vi "TH2829_Analysis_Data.vi"(0 "字符串":string) -> (14 "Turns Result":sgl[][](array[numeric]) format="%#_6f", 15 "Lx Result":sgl[][](array[numeric]) format="%#_6f", 16 "Lk Result":sgl[][](array[numeric]) format="%#_6f", 17 "DCR Result":sgl[][](array[numeric]) format="%#_6f")   [LabVIEW 2018]
panel:
  out "LED IrCompare Result":u8[][](array[numeric])
  out "LED VfCompare Result":u8[][](array[numeric])
  out "LED IrResult":sgl[][](array[numeric]) format="%#_6f"
  out "LED VfResult":sgl[][](array[numeric]) format="%#_6f"
  out "Bls Result":sgl[][](array[numeric]) format="%#_6f"
  out "总判断":u8
  out "PS Compare Result":u8[][](array[numeric])
  out "Balance Compare Result":u8[][](array[numeric])
  out "Z Compare Result":u8[][](array[numeric])
  out "Rs Compare Result":u8[][](array[numeric])
  out "LxQ Compare Result":u8[][](array[numeric])
  out "DCR Compare Result":u8[][](array[numeric])
  out "C Compare Result":u8[][](array[numeric])
  out "Lk Compare Result":u8[][](array[numeric])
  out "Lx Compare Result":u8[][](array[numeric])
  out "Turns Compare Result":u8[][](array[numeric])
  out "Polarity Result1":string[][](array[string])
  out "Polarity Result":u8[][](array[numeric])
  out "Zx Result":sgl[][](array[numeric]) format="%#_6f"
  out "ACR Result":sgl[][](array[numeric]) format="%#_6f"
  out "LxQ Result":sgl[][](array[numeric]) format="%#_6f"
  out "Cx Result":sgl[][](array[numeric]) format="%#_6f"
  out "Primary Sets":string
  out "head":string
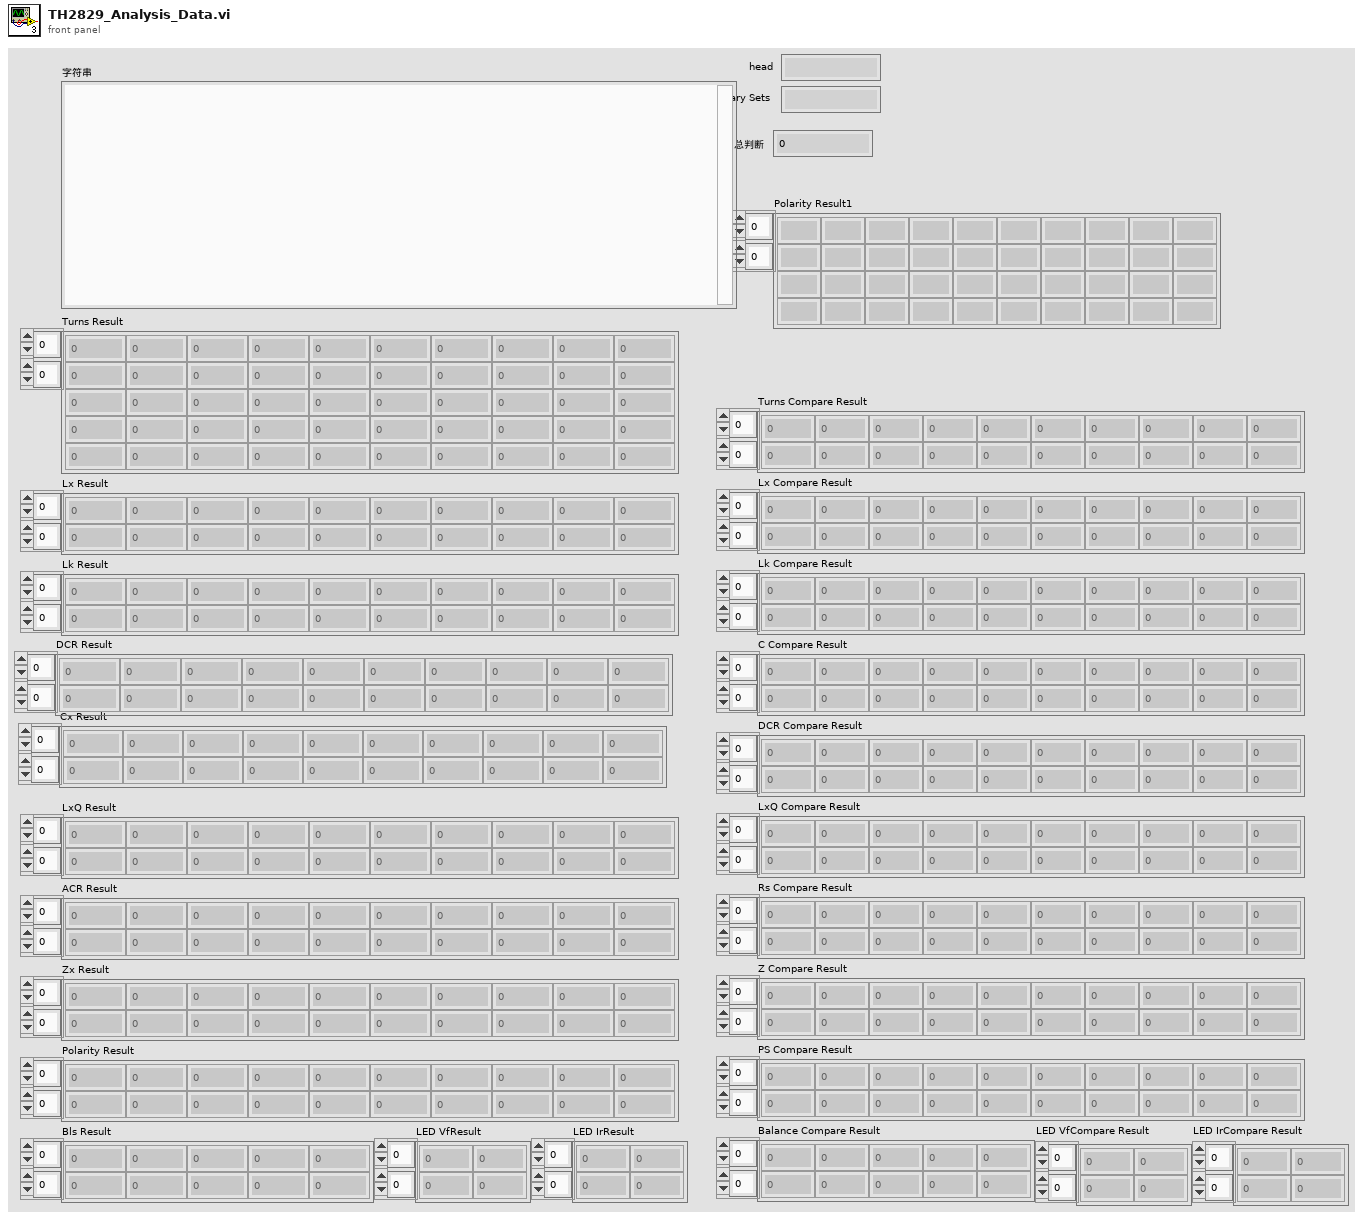
[diagram p1: front panel]
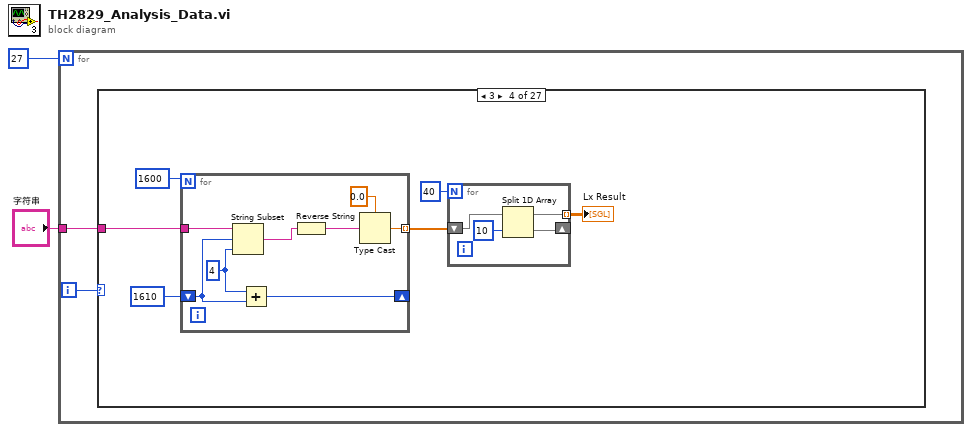
[diagram p0: block diagram]
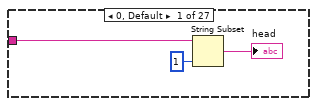
[diagram p2: hidden frame]
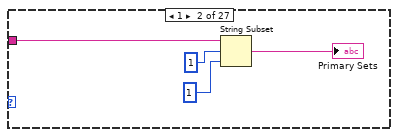
[diagram p3: hidden frame]
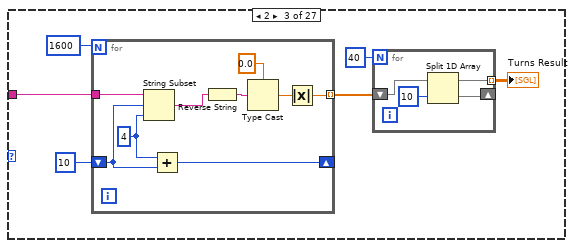
[diagram p4: hidden frame]
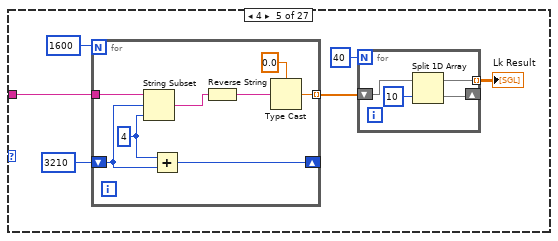
[diagram p5: hidden frame]
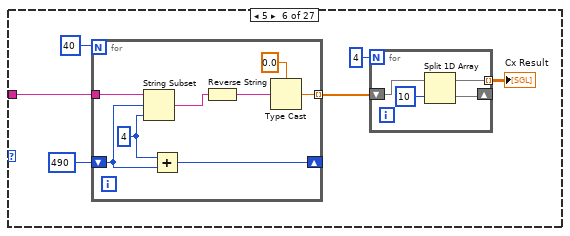
[diagram p6: hidden frame]
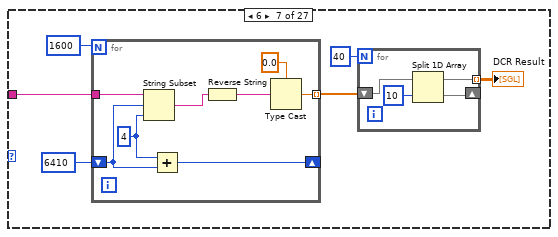
[diagram p7: hidden frame]
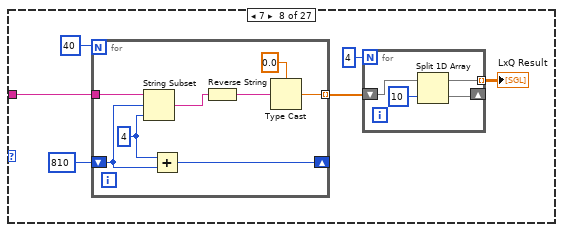
[diagram p8: hidden frame]
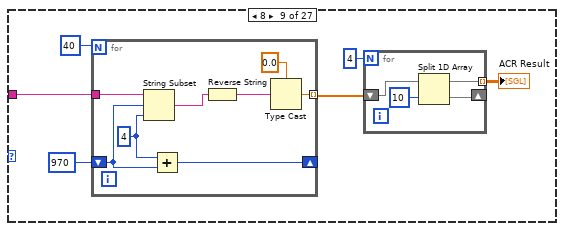
[diagram p9: hidden frame]
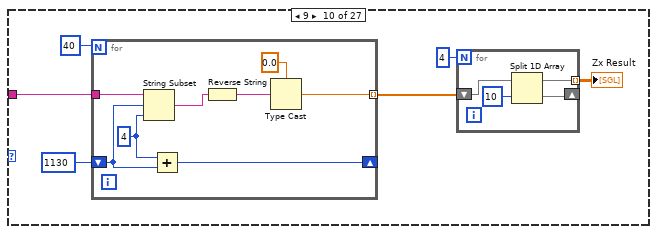
[diagram p10: hidden frame]
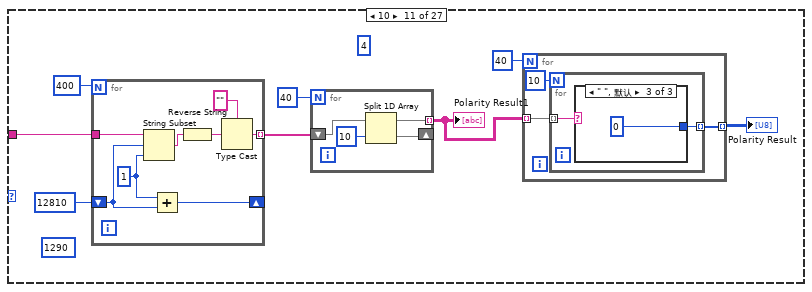
[diagram p11: hidden frame]
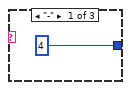
[diagram p12: hidden frame]
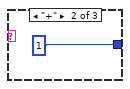
[diagram p13: hidden frame]
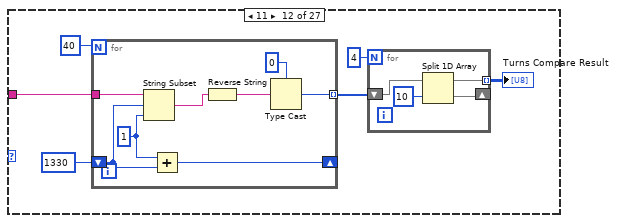
[diagram p14: hidden frame]
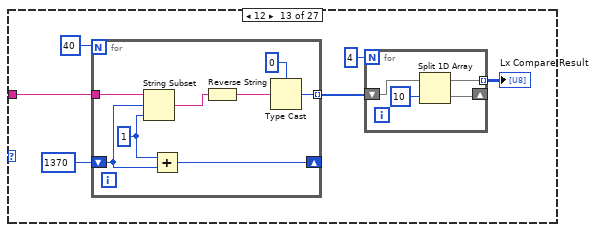
[diagram p15: hidden frame]
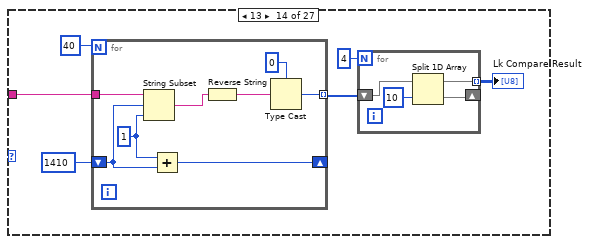
[diagram p16: hidden frame]
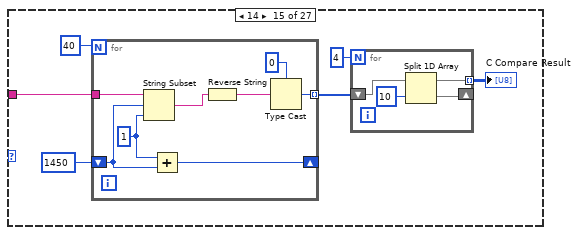
[diagram p17: hidden frame]
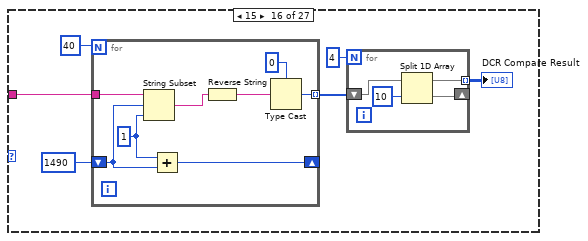
[diagram p18: hidden frame]
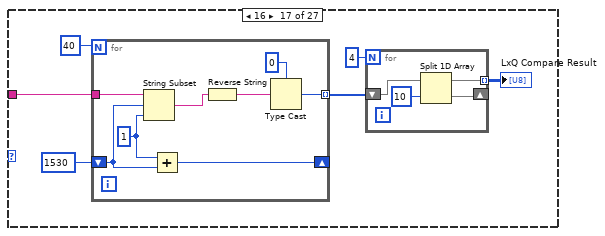
[diagram p19: hidden frame]
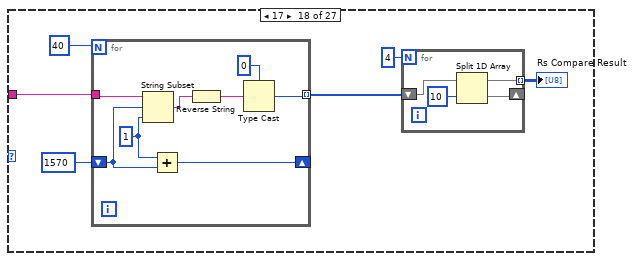
[diagram p20: hidden frame]
diagram:
  n1 = for {
    N: 27 -> [_]
    tunnel: "字符串" -> [w3]
    i -> [w4]
    n2 = case shown="3" w4 {
      tunnel: w3 -> [w7 w11 w16 w35 w53 w71 w89 w107 w125 w143 w163 w189 w207 w225 w243 w261 w279 w297 w315 w333 w351 w368 w372 w390 w408 w426 w444]
      frame 0, Default {
        n3 = String Subset(string=w7, length (rest)=1 ("长度（剩余）")) -> (substring=→"head":string)  [unwired: 1 in]
      }
      frame 1 {
        n4 = String Subset ("截取字符串")(string=w11, offset (0)=1 ("长度（剩余）"), length (rest)=1 ("长度（剩余）")) -> (substring=→"Primary Sets":string)
      }
      frame 2 {
        n5 = for {
          N: 1600 -> [_]
          shift-right: [w26] -> _
          shift-left: 10 ("长度（剩余）") -> [w22]
          tunnel: w16 -> [w21]
          tunnel: [w18] -> w14 mode=indexing
          w23 = 4 ("长度（剩余）")
          n6 = String Subset(string=w21, offset (0)=w22, length (rest)=w23) -> (substring=w20:string)
          n7 = Add(x=w23, y=w22) -> (x+y=w26:i32)
          n8 = Reverse String(1:w20) -> (0:w25:string)
          n9 = Type Cast(type=sgl 0.0 ("长度（剩余）"), x=w25) -> (*(type *) &x=w19:sgl)
          n10 = Absolute Value(x=w19) -> (abs(x)=w18:sgl)
        }
        n11 = for {
          N: 40 -> [_]
          shift-right: [w29] -> _
          shift-left: w14 -> [w27]
          tunnel: [w28] -> w12 mode=indexing
          n12 = Split 1D Array(array=w27, index=10 ("索引")) -> (first subarray=w28:sgl[], second subarray=w29:sgl[])
        }
        "Turns Result" <- w12
      }
      frame 3 {
        n13 = for {
          N: 1600 -> [_]
          shift-right: [w44] -> _
          shift-left: 1610 ("长度（剩余）") -> [w40]
          tunnel: w35 -> [w39]
          tunnel: [w37] -> w33 mode=indexing
          w41 = 4 ("长度（剩余）")
          n14 = String Subset(string=w39, offset (0)=w40, length (rest)=w41) -> (substring=w38:string)
          n15 = Add(x=w41, y=w40) -> (x+y=w44:i32)
          n16 = Reverse String(1:w38) -> (0:w43:string)
          n17 = Type Cast(type=sgl 0.0 ("长度（剩余）"), x=w43) -> (*(type *) &x=w37:sgl)
        }
        n18 = for {
          N: 40 -> [_]
          shift-right: [w47] -> _
          shift-left: w33 -> [w45]
          tunnel: [w46] -> w31 mode=indexing
          n19 = Split 1D Array(array=w45, index=10 ("索引")) -> (first subarray=w46:sgl[], second subarray=w47:sgl[])
        }
        "Lx Result" <- w31
      }
      frame 4 {
        n20 = for {
          N: 1600 -> [_]
          shift-right: [w62] -> _
          shift-left: 3210 ("长度（剩余）") -> [w58]
          tunnel: w53 -> [w57]
          tunnel: [w55] -> w51 mode=indexing
          w59 = 4 ("长度（剩余）")
          n21 = String Subset(string=w57, offset (0)=w58, length (rest)=w59) -> (substring=w56:string)
          n22 = Add(x=w59, y=w58) -> (x+y=w62:i32)
          n23 = Reverse String(1:w56) -> (0:w61:string)
          n24 = Type Cast(type=sgl 0.0 ("长度（剩余）"), x=w61) -> (*(type *) &x=w55:sgl)
        }
        n25 = for {
          N: 40 -> [_]
          shift-right: [w65] -> _
          shift-left: w51 -> [w63]
          tunnel: [w64] -> w49 mode=indexing
          n26 = Split 1D Array(array=w63, index=10 ("索引")) -> (first subarray=w64:sgl[], second subarray=w65:sgl[])
        }
        "Lk Result" <- w49
      }
      frame 5 {
        n27 = for {
          N: 40 -> [_]
          shift-right: [w80] -> _
          shift-left: 490 ("长度（剩余）") -> [w76]
          tunnel: w71 -> [w75]
          tunnel: [w73] -> w69 mode=indexing
          w77 = 4 ("长度（剩余）")
          n28 = String Subset(string=w75, offset (0)=w76, length (rest)=w77) -> (substring=w74:string)
          n29 = Add(x=w77, y=w76) -> (x+y=w80:i32)
          n30 = Reverse String(1:w74) -> (0:w79:string)
          n31 = Type Cast(type=sgl 0.0 ("长度（剩余）"), x=w79) -> (*(type *) &x=w73:sgl)
        }
        n32 = for {
          N: 4 -> [_]
          shift-right: [w83] -> _
          shift-left: w69 -> [w81]
          tunnel: [w82] -> w67 mode=indexing
          n33 = Split 1D Array(array=w81, index=10 ("索引")) -> (first subarray=w82:sgl[], second subarray=w83:sgl[])
        }
        "Cx Result" <- w67
      }
      frame 6 {
        n34 = for {
          N: 1600 -> [_]
          shift-right: [w98] -> _
          shift-left: 6410 ("长度（剩余）") -> [w94]
          tunnel: w89 -> [w93]
          tunnel: [w91] -> w87 mode=indexing
          w95 = 4 ("长度（剩余）")
          n35 = String Subset(string=w93, offset (0)=w94, length (rest)=w95) -> (substring=w92:string)
          n36 = Add(x=w95, y=w94) -> (x+y=w98:i32)
          n37 = Reverse String(1:w92) -> (0:w97:string)
          n38 = Type Cast(type=sgl 0.0 ("长度（剩余）"), x=w97) -> (*(type *) &x=w91:sgl)
        }
        n39 = for {
          N: 40 -> [_]
          shift-right: [w101] -> _
          shift-left: w87 -> [w99]
          tunnel: [w100] -> w85 mode=indexing
          n40 = Split 1D Array(array=w99, index=10 ("索引")) -> (first subarray=w100:sgl[], second subarray=w101:sgl[])
        }
        "DCR Result" <- w85
      }
      frame 7 {
        n41 = for {
          N: 40 -> [_]
          shift-right: [w116] -> _
          shift-left: 810 ("长度（剩余）") -> [w112]
          tunnel: w107 -> [w111]
          tunnel: [w109] -> w105 mode=indexing
          w113 = 4 ("长度（剩余）")
          n42 = String Subset(string=w111, offset (0)=w112, length (rest)=w113) -> (substring=w110:string)
          n43 = Add(x=w113, y=w112) -> (x+y=w116:i32)
          n44 = Reverse String(1:w110) -> (0:w115:string)
          n45 = Type Cast(type=sgl 0.0 ("长度（剩余）"), x=w115) -> (*(type *) &x=w109:sgl)
        }
        n46 = for {
          N: 4 -> [_]
          shift-right: [w119] -> _
          shift-left: w105 -> [w117]
          tunnel: [w118] -> w103 mode=indexing
          n47 = Split 1D Array(array=w117, index=10 ("索引")) -> (first subarray=w118:sgl[], second subarray=w119:sgl[])
        }
        "LxQ Result" <- w103
      }
      frame 8 {
        n48 = for {
          N: 40 -> [_]
          shift-right: [w134] -> _
          shift-left: 970 ("长度（剩余）") -> [w130]
          tunnel: w125 -> [w129]
          tunnel: [w127] -> w123 mode=indexing
          w131 = 4 ("长度（剩余）")
          n49 = String Subset(string=w129, offset (0)=w130, length (rest)=w131) -> (substring=w128:string)
          n50 = Add(x=w131, y=w130) -> (x+y=w134:i32)
          n51 = Reverse String(1:w128) -> (0:w133:string)
          n52 = Type Cast(type=sgl 0.0 ("长度（剩余）"), x=w133) -> (*(type *) &x=w127:sgl)
        }
        n53 = for {
          N: 4 -> [_]
          shift-right: [w137] -> _
          shift-left: w123 -> [w135]
          tunnel: [w136] -> w121 mode=indexing
          n54 = Split 1D Array(array=w135, index=10 ("索引")) -> (first subarray=w136:sgl[], second subarray=w137:sgl[])
        }
        "ACR Result" <- w121
      }
      frame 9 {
        n55 = for {
          N: 40 -> [_]
          shift-right: [w152] -> _
          shift-left: 1130 ("长度（剩余）") -> [w148]
          tunnel: w143 -> [w147]
          tunnel: [w145] -> w141 mode=indexing
          w149 = 4 ("长度（剩余）")
          n56 = String Subset(string=w147, offset (0)=w148, length (rest)=w149) -> (substring=w146:string)
          n57 = Add(x=w149, y=w148) -> (x+y=w152:i32)
          n58 = Reverse String(1:w146) -> (0:w151:string)
          n59 = Type Cast(type=sgl 0.0 ("长度（剩余）"), x=w151) -> (*(type *) &x=w145:sgl)
        }
        n60 = for {
          N: 4 -> [_]
          shift-right: [w155] -> _
          shift-left: w141 -> [w153]
          tunnel: [w154] -> w139 mode=indexing
          n61 = Split 1D Array(array=w153, index=10 ("索引")) -> (first subarray=w154:sgl[], second subarray=w155:sgl[])
        }
        "Zx Result" <- w139
      }
      frame 10 {
        (unwired) 1290 ("长度（剩余）")
        (unwired) 4
        n62 = for {
          N: 400 -> [_]
          shift-right: [w180] -> _
          shift-left: 12810 ("长度（剩余）") -> [w177]
          tunnel: w163 -> [w176]
          tunnel: [w174] -> w158 mode=indexing
          w178 = 1 ("长度（剩余）")
          n63 = String Subset(string=w176, offset (0)=w177, length (rest)=w178) -> (substring=w175:string)
          n64 = Add(x=w178, y=w177) -> (x+y=w180:i32)
          n65 = Reverse String(1:w175) -> (0:w179:string)
          n66 = Type Cast(type="", x=w179) -> (*(type *) &x=w174:string)
        }
        n67 = for {
          N: 40 -> [_]
          shift-right: [w183] -> _
          shift-left: w158 -> [w181]
          tunnel: [w182] -> w157 mode=indexing
          n68 = Split 1D Array(array=w181, index=10 ("索引")) -> (first subarray=w182:string[], second subarray=w183:string[])
        }
        "Polarity Result1" <- w157
        n69 = for {
          N: 40 -> [_]
          tunnel: w157 -> [w166] mode=indexing
          tunnel: [w165] -> w159 mode=indexing
          n70 = for {
            N: 10 -> [_]
            tunnel: w166 -> [w169] mode=indexing
            tunnel: [w168] -> w165 mode=indexing
            n71 = case shown="\" \", 默认" w169 {
              tunnel: [u8 4 u8 1 u8 0] -> w168
              frame "-" {
              }
              frame "+" {
              }
              frame " ", Default {
              }
            }
          }
        }
        "Polarity Result" <- w159
      }
      frame 11 {
        n72 = for {
          N: 40 -> [_]
          shift-right: [w198] -> _
          shift-left: 1330 ("长度（剩余）") -> [w194]
          tunnel: w189 -> [w193]
          tunnel: [w191] -> w187 mode=indexing
          w195 = 1 ("长度（剩余）")
          n73 = String Subset ("截取字符串")(string=w193, offset (0)=w194, length (rest)=w195) -> (substring=w192:string)
          n74 = Add(x=w195, y=w194) -> (x+y=w198:i32)
          n75 = Reverse String(1:w192) -> (0:w197:string)
          n76 = Type Cast(type=u8 0 ("长度（剩余）"), x=w197) -> (*(type *) &x=w191:u8)
        }
        n77 = for {
          N: 4 -> [_]
          shift-right: [w201] -> _
          shift-left: w187 -> [w199]
          tunnel: [w200] -> w185 mode=indexing
          n78 = Split 1D Array(array=w199, index=10 ("索引")) -> (first subarray=w200:u8[], second subarray=w201:u8[])
        }
        "Turns Compare Result" <- w185
      }
      frame 12 {
        n79 = for {
          N: 40 -> [_]
          shift-right: [w216] -> _
          shift-left: 1370 ("长度（剩余）") -> [w212]
          tunnel: w207 -> [w211]
          tunnel: [w209] -> w205 mode=indexing
          w213 = 1 ("长度（剩余）")
          n80 = String Subset(string=w211, offset (0)=w212, length (rest)=w213) -> (substring=w210:string)
          n81 = Add(x=w213, y=w212) -> (x+y=w216:i32)
          n82 = Reverse String(1:w210) -> (0:w215:string)
          n83 = Type Cast(type=u8 0 ("长度（剩余）"), x=w215) -> (*(type *) &x=w209:u8)
        }
        n84 = for {
          N: 4 -> [_]
          shift-right: [w219] -> _
          shift-left: w205 -> [w217]
          tunnel: [w218] -> w203 mode=indexing
          n85 = Split 1D Array(array=w217, index=10 ("索引")) -> (first subarray=w218:u8[], second subarray=w219:u8[])
        }
        "Lx Compare Result" <- w203
      }
      frame 13 {
        n86 = for {
          N: 40 -> [_]
          shift-right: [w234] -> _
          shift-left: 1410 ("长度（剩余）") -> [w230]
          tunnel: w225 -> [w229]
          tunnel: [w227] -> w223 mode=indexing
          w231 = 1 ("长度（剩余）")
          n87 = String Subset(string=w229, offset (0)=w230, length (rest)=w231) -> (substring=w228:string)
          n88 = Add(x=w231, y=w230) -> (x+y=w234:i32)
          n89 = Reverse String(1:w228) -> (0:w233:string)
          n90 = Type Cast(type=u8 0 ("长度（剩余）"), x=w233) -> (*(type *) &x=w227:u8)
        }
        n91 = for {
          N: 4 -> [_]
          shift-right: [w237] -> _
          shift-left: w223 -> [w235]
          tunnel: [w236] -> w221 mode=indexing
          n92 = Split 1D Array(array=w235, index=10 ("索引")) -> (first subarray=w236:u8[], second subarray=w237:u8[])
        }
        "Lk Compare Result" <- w221
      }
      frame 14 {
        n93 = for {
          N: 40 -> [_]
          shift-right: [w252] -> _
          shift-left: 1450 ("长度（剩余）") -> [w248]
          tunnel: w243 -> [w247]
          tunnel: [w245] -> w241 mode=indexing
          w249 = 1 ("长度（剩余）")
          n94 = String Subset(string=w247, offset (0)=w248, length (rest)=w249) -> (substring=w246:string)
          n95 = Add(x=w249, y=w248) -> (x+y=w252:i32)
          n96 = Reverse String(1:w246) -> (0:w251:string)
          n97 = Type Cast(type=u8 0 ("长度（剩余）"), x=w251) -> (*(type *) &x=w245:u8)
        }
        n98 = for {
          N: 4 -> [_]
          shift-right: [w255] -> _
          shift-left: w241 -> [w253]
          tunnel: [w254] -> w239 mode=indexing
          n99 = Split 1D Array(array=w253, index=10 ("索引")) -> (first subarray=w254:u8[], second subarray=w255:u8[])
        }
        "C Compare Result" <- w239
      }
      frame 15 {
        n100 = for {
          N: 40 -> [_]
          shift-right: [w270] -> _
          shift-left: 1490 ("长度（剩余）") -> [w266]
          tunnel: w261 -> [w265]
          tunnel: [w263] -> w259 mode=indexing
          w267 = 1 ("长度（剩余）")
          n101 = String Subset(string=w265, offset (0)=w266, length (rest)=w267) -> (substring=w264:string)
          n102 = Add(x=w267, y=w266) -> (x+y=w270:i32)
          n103 = Reverse String(1:w264) -> (0:w269:string)
          n104 = Type Cast(type=u8 0 ("长度（剩余）"), x=w269) -> (*(type *) &x=w263:u8)
        }
        n105 = for {
          N: 4 -> [_]
          shift-right: [w273] -> _
          shift-left: w259 -> [w271]
          tunnel: [w272] -> w257 mode=indexing
          n106 = Split 1D Array(array=w271, index=10 ("索引")) -> (first subarray=w272:u8[], second subarray=w273:u8[])
        }
        "DCR Compare Result" <- w257
      }
      frame 16 {
        n107 = for {
          N: 40 -> [_]
          shift-right: [w288] -> _
          shift-left: 1530 ("长度（剩余）") -> [w284]
          tunnel: w279 -> [w283]
          tunnel: [w281] -> w277 mode=indexing
          w285 = 1 ("长度（剩余）")
          n108 = String Subset(string=w283, offset (0)=w284, length (rest)=w285) -> (substring=w282:string)
          n109 = Add(x=w285, y=w284) -> (x+y=w288:i32)
          n110 = Reverse String(1:w282) -> (0:w287:string)
          n111 = Type Cast(type=u8 0 ("长度（剩余）"), x=w287) -> (*(type *) &x=w281:u8)
        }
        n112 = for {
          N: 4 -> [_]
          shift-right: [w291] -> _
          shift-left: w277 -> [w289]
          tunnel: [w290] -> w275 mode=indexing
          n113 = Split 1D Array(array=w289, index=10 ("索引")) -> (first subarray=w290:u8[], second subarray=w291:u8[])
        }
        "LxQ Compare Result" <- w275
      }
      frame 17 {
        n114 = for {
          N: 40 -> [_]
          shift-right: [w306] -> _
          shift-left: 1570 ("长度（剩余）") -> [w300]
          tunnel: w297 -> [w301]
          tunnel: [w302] -> w295 mode=indexing
          w299 = 1 ("长度（剩余）")
          n115 = String Subset(string=w301, offset (0)=w300, length (rest)=w299) -> (substring=w303:string)
          n116 = Add(x=w299, y=w300) -> (x+y=w306:i32)
          n117 = Reverse String(1:w303) -> (0:w305:string)
          n118 = Type Cast(type=u8 0 ("长度（剩余）"), x=w305) -> (*(type *) &x=w302:u8)
        }
        n119 = for {
          N: 4 -> [_]
          shift-right: [w309] -> _
          shift-left: w295 -> [w307]
          tunnel: [w308] -> w293 mode=indexing
          n120 = Split 1D Array(array=w307, index=10 ("索引")) -> (first subarray=w308:u8[], second subarray=w309:u8[])
        }
        "Rs Compare Result" <- w293
      }
      frame 18 {
        n121 = for {
          N: 40 -> [_]
          shift-right: [w324] -> _
          shift-left: 1610 ("长度（剩余）") -> [w318]
          tunnel: w315 -> [w319]
          tunnel: [w320] -> w313 mode=indexing
          w317 = 1 ("长度（剩余）")
          n122 = Add(x=w317, y=w318) -> (x+y=w324:i32)
          n123 = String Subset(string=w319, offset (0)=w318, length (rest)=w317) -> (substring=w321:string)
          n124 = Reverse String(1:w321) -> (0:w323:string)
          n125 = Type Cast(type=u8 0 ("长度（剩余）"), x=w323) -> (*(type *) &x=w320:u8)
        }
        n126 = for {
          N: 4 -> [_]
          shift-right: [w327] -> _
          shift-left: w313 -> [w325]
          tunnel: [w326] -> w311 mode=indexing
          n127 = Split 1D Array(array=w325, index=10 ("索引")) -> (first subarray=w326:u8[], second subarray=w327:u8[])
        }
        "Z Compare Result" <- w311
      }
      frame 19 {
        n128 = for {
          N: 40 -> [_]
          shift-right: [w342] -> _
          shift-left: 1650 ("长度（剩余）") -> [w337]
          tunnel: w333 -> [w338]
          tunnel: [w339] -> w331 mode=indexing
          w336 = 1 ("长度（剩余）")
          n129 = String Subset(string=w338, offset (0)=w337, length (rest)=w336) -> (substring=w340:string)
          n130 = Add(x=w336, y=w337) -> (x+y=w342:i32)
          n131 = Reverse String(1:w340) -> (0:w341:string)
          n132 = Type Cast(type=u8 0 ("长度（剩余）"), x=w341) -> (*(type *) &x=w339:u8)
        }
        n133 = for {
          N: 4 -> [_]
          shift-right: [w345] -> _
          shift-left: w331 -> [w343]
          tunnel: [w344] -> w329 mode=indexing
          n134 = Split 1D Array(array=w343, index=10 ("索引")) -> (first subarray=w344:u8[], second subarray=w345:u8[])
        }
        "Balance Compare Result" <- w329
      }
      frame 20 {
        n135 = for {
          N: 40 -> [_]
          shift-right: [w360] -> _
          shift-left: 1690 ("长度（剩余）") -> [w355]
          tunnel: w351 -> [w356]
          tunnel: [w357] -> w349 mode=indexing
          w354 = 1 ("长度（剩余）")
          n136 = String Subset(string=w356, offset (0)=w355, length (rest)=w354) -> (substring=w358:string)
          n137 = Add(x=w354, y=w355) -> (x+y=w360:i32)
          n138 = Reverse String(1:w358) -> (0:w359:string)
          n139 = Type Cast(type=u8 0 ("长度（剩余）"), x=w359) -> (*(type *) &x=w357:u8)
        }
        n140 = for {
          N: 4 -> [_]
          shift-right: [w363] -> _
          shift-left: w349 -> [w361]
          tunnel: [w362] -> w347 mode=indexing
          n141 = Split 1D Array(array=w361, index=10 ("索引")) -> (first subarray=w362:u8[], second subarray=w363:u8[])
        }
        "PS Compare Result" <- w347
      }
      frame 21 {
        n142 = String Subset(string=w368, offset (0)=1730 ("长度（剩余）"), length (rest)=1 ("长度（剩余）")) -> (substring=w371:string)
        n143 = Reverse String(1:w371) -> (0:w369:string)
        n144 = Type Cast(type=u8 0 ("长度（剩余）"), x=w369) -> (*(type *) &x=→"总判断":u8)
      }
      frame 22 {
        n145 = for {
          N: 20 -> [_]
          shift-right: [w385] -> _
          shift-left: 1731 ("长度（剩余）") -> [w381]
          tunnel: w372 -> [w380]
          tunnel: [w378] -> w375 mode=indexing
          w382 = 4 ("长度（剩余）")
          n146 = String Subset(string=w380, offset (0)=w381, length (rest)=w382) -> (substring=w379:string)
          n147 = Add(x=w382, y=w381) -> (x+y=w385:i32)
          n148 = Reverse String(1:w379) -> (0:w384:string)
          n149 = Type Cast(type=sgl 0.0 ("长度（剩余）"), x=w384) -> (*(type *) &x=w378:sgl)
        }
        n150 = for {
          N: 4 -> [_]
          shift-right: [w388] -> _
          shift-left: w375 -> [w386]
          tunnel: [w387] -> w373 mode=indexing
          n151 = Split 1D Array(array=w386, index=5 ("索引")) -> (first subarray=w387:sgl[], second subarray=w388:sgl[])
        }
        "Bls Result" <- w373
      }
      frame 23 {
        n152 = for {
          N: 8 -> [_]
          shift-right: [w403] -> _
          shift-left: 1811 ("长度（剩余）") -> [w399]
          tunnel: w390 -> [w398]
          tunnel: [w396] -> w392 mode=indexing
          w400 = 4 ("长度（剩余）")
          n153 = String Subset(string=w398, offset (0)=w399, length (rest)=w400) -> (substring=w397:string)
          n154 = Add(x=w400, y=w399) -> (x+y=w403:i32)
          n155 = Reverse String(1:w397) -> (0:w402:string)
          n156 = Type Cast(type=sgl 0.0 ("长度（剩余）"), x=w402) -> (*(type *) &x=w396:sgl)
        }
        n157 = for {
          N: 4 -> [_]
          shift-right: [w406] -> _
          shift-left: w392 -> [w404]
          tunnel: [w405] -> w395 mode=indexing
          n158 = Split 1D Array(array=w404, index=2 ("索引")) -> (first subarray=w405:sgl[], second subarray=w406:sgl[])
        }
        "LED VfResult" <- w395
      }
      frame 24 {
        n159 = for {
          N: 8 -> [_]
          shift-right: [w421] -> _
          shift-left: 1843 ("长度（剩余）") -> [w417]
          tunnel: w408 -> [w416]
          tunnel: [w414] -> w410 mode=indexing
          w418 = 4 ("长度（剩余）")
          n160 = String Subset(string=w416, offset (0)=w417, length (rest)=w418) -> (substring=w415:string)
          n161 = Add(x=w418, y=w417) -> (x+y=w421:i32)
          n162 = Reverse String(1:w415) -> (0:w420:string)
          n163 = Type Cast(type=sgl 0.0 ("长度（剩余）"), x=w420) -> (*(type *) &x=w414:sgl)
        }
        n164 = for {
          N: 4 -> [_]
          shift-right: [w424] -> _
          shift-left: w410 -> [w422]
          tunnel: [w423] -> w413 mode=indexing
          n165 = Split 1D Array(array=w422, index=2 ("索引")) -> (first subarray=w423:sgl[], second subarray=w424:sgl[])
        }
        "LED IrResult" <- w413
      }
      frame 25 {
        n166 = for {
          N: 8 -> [_]
          shift-right: [w439] -> _
          shift-left: 1875 ("长度（剩余）") -> [w434]
          tunnel: w426 -> [w435]
          tunnel: [w436] -> w428 mode=indexing
          w433 = 1 ("长度（剩余）")
          n167 = String Subset(string=w435, offset (0)=w434, length (rest)=w433) -> (substring=w437:string)
          n168 = Add(x=w433, y=w434) -> (x+y=w439:i32)
          n169 = Reverse String(1:w437) -> (0:w438:string)
          n170 = Type Cast(type=u8 0 ("长度（剩余）"), x=w438) -> (*(type *) &x=w436:u8)
        }
        n171 = for {
          N: 4 -> [_]
          shift-right: [w442] -> _
          shift-left: w428 -> [w440]
          tunnel: [w441] -> w431 mode=indexing
          n172 = Split 1D Array(array=w440, index=2 ("索引")) -> (first subarray=w441:u8[], second subarray=w442:u8[])
        }
        "LED VfCompare Result" <- w431
      }
      frame 26 {
        n173 = for {
          N: 8 -> [_]
          shift-right: [w457] -> _
          shift-left: 1883 ("长度（剩余）") -> [w452]
          tunnel: w444 -> [w453]
          tunnel: [w454] -> w446 mode=indexing
          w451 = 1 ("长度（剩余）")
          n174 = String Subset(string=w453, offset (0)=w452, length (rest)=w451) -> (substring=w455:string)
          n175 = Add(x=w451, y=w452) -> (x+y=w457:i32)
          n176 = Reverse String(1:w455) -> (0:w456:string)
          n177 = Type Cast(type=u8 0 ("长度（剩余）"), x=w456) -> (*(type *) &x=w454:u8)
        }
        n178 = for {
          N: 4 -> [_]
          shift-right: [w460] -> _
          shift-left: w446 -> [w458]
          tunnel: [w459] -> w449 mode=indexing
          n179 = Split 1D Array(array=w458, index=2 ("索引")) -> (first subarray=w459:u8[], second subarray=w460:u8[])
        }
        "LED IrCompare Result" <- w449
      }
    }
  }
